vi "DrawTraveledPath.vi"(8 "error in (no error)":errorcluster, 9 "end point":cluster{"x":i16, "y":i16}, 10 "start point":cluster{"x":i16, "y":i16}, 11 "picture":picture) -> (0 "error out":errorcluster, 3 "new picture":picture)   [LabVIEW 2009, in "Host.lvlib" / "Draw.lvlib"]
uses:
  Draw.lvlib
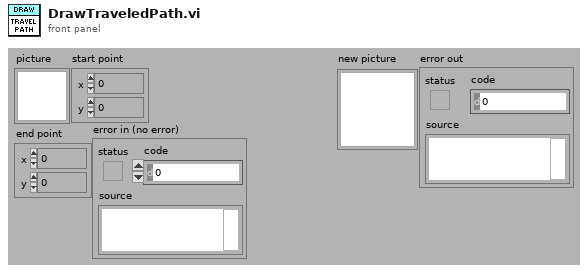
[diagram p1: front panel]
types:
  T1 = cluster{"Width":u16, "Style":enum32{"Solid", "Dash", "Dot", "DashDot", "DashDotDot"}}
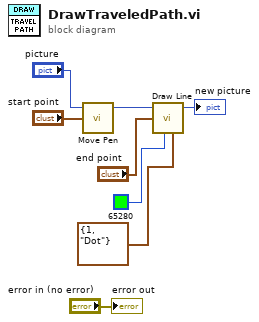
[diagram p0: block diagram]
diagram:
  n1 = call <vilib>:"Move Pen.vi"("new position"="start point", "picture"="picture") -> ("new picture"=w7:picture)  [unwired: 3 in]
  n2 = call <vilib>:"Draw Line.vi"("picture"=w7, "end point"="end point", "color(black)"=u32 65280, "pen"=T1 {"Width"=1, "Style"=enum."Dot"}) -> ("new picture"=→"new picture":picture)  [unwired: 5 in]
  "error out" <- "error in (no error)"
